vi "Get Array Element Offsets.vi"(8 "error in (no error)":errorcluster, 9 "Max Index":i32=2147483647, 10 "Offset":i32, 11 "JSON":string) -> (0 "error out":errorcluster, 1 "Elements":T2(array[cluster]), 2 "Offset past Array":i32)   [LabVIEW 2017, in "JSONtext.lvlib"]
uses:
  JSONtext.lvlib
  Parsing/Parsing State.ctl
  Parsing/Advance past String.vi
  Parsing/Advance past Number.vi
  Parsing/Advance past Object.vi
  Parsing/Advance past Array.vi
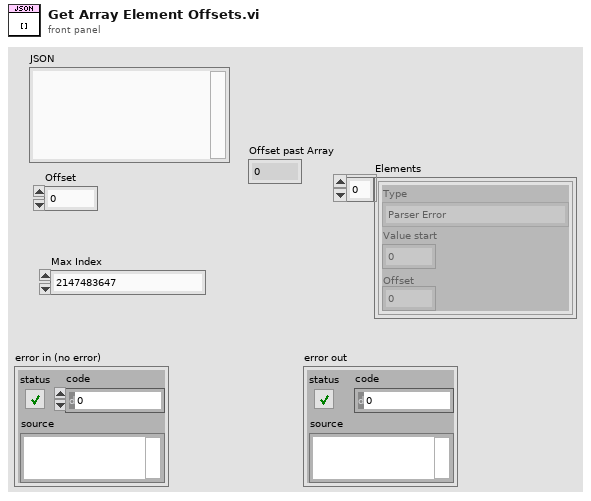
[diagram p1: front panel]
types:
  T1 = typedef "JSONtext.lvlib/Parsing State.ctl" = enum16{"Parser Error", "Object", "Array", "String", "Number/Other", "Leading Whitespace", "Object end", "Array end", "Value end"}
  T2 = cluster{"Type":T1, "Value start":i32, "Offset":i32}[]
  T3 = cluster{"Type":T1, "Value start":i32, "Offset":i32}
  T4 = cluster{"State":T1, "Value start":i32, "index":i32}
  T5 = cluster{"State":T1, "Value start":i32, "index":i32}[]
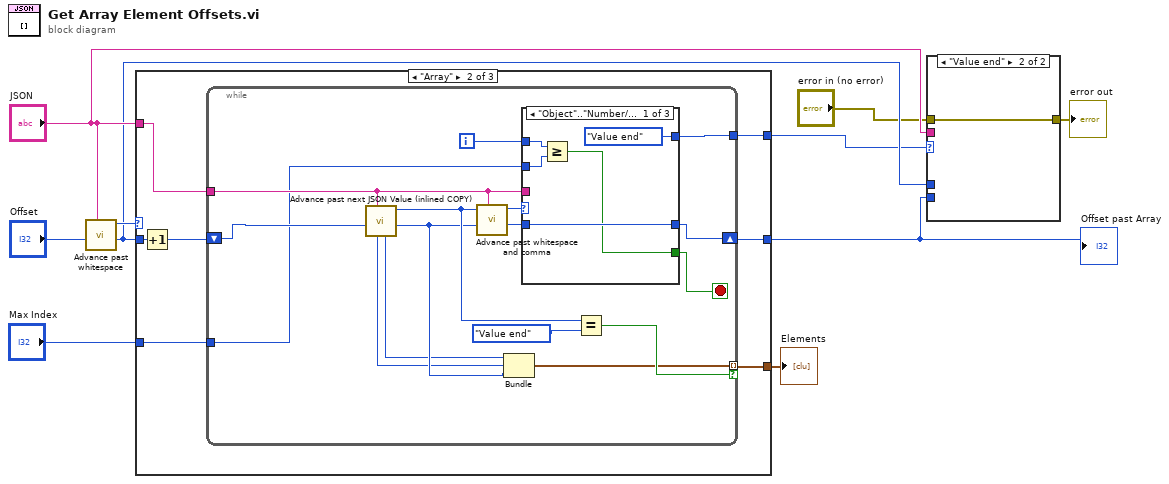
[diagram p0: block diagram]
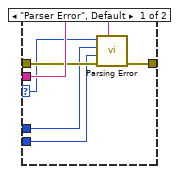
[diagram p2: hidden frame]
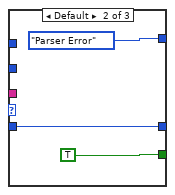
[diagram p4: hidden frame]
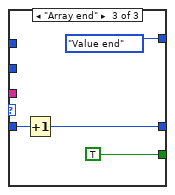
[diagram p5: hidden frame]
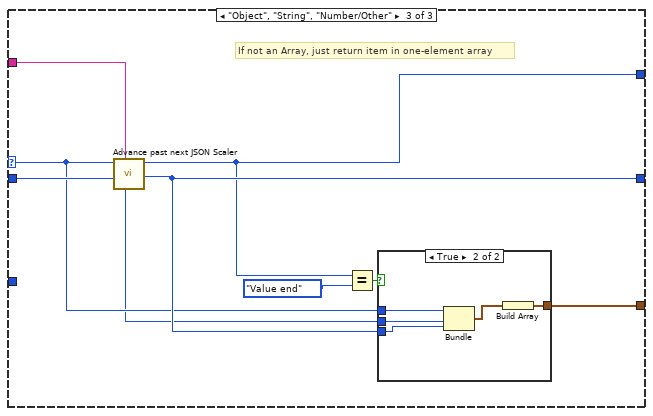
[diagram p6: hidden frame]
diagram:
  n1 = call "Advance past whitespace.vi"("JSON"="JSON", "Offset"="Offset") -> ("Offset of first non-whitespace"=w7:i32, "Parser State"=w9:T1)  [unwired: 8 in]
  n2 = case shown="\"Array\"" w9 {
    selector: w9 -> [w12 _ w50]
    tunnel: [w12 w19 w52] -> w3
    tunnel: [w11 w18 w54] -> w6
    tunnel: [_ w16 w49] -> w2
    tunnel: "JSON" -> [_ w15 w53]
    tunnel: w7 -> [w11 w14 w56]
    tunnel: "Max Index" -> [_ w13 _]
    frame "Parser Error", Default {
    }
    frame "Array" {
      n3 = Increment(x=w14) -> (x+1=w17:i32)
      n4 = while {
        tunnel: w15 -> [w29]
        shift-right: [w32] -> w18
        shift-left: w17 -> [w33]
        tunnel: [w30] -> w19
        tunnel: [w23] -> w16 mode=indexing if=w26
        tunnel: w13 -> [w20]
        i -> [w21]
        stop <- w31 stop-if-true
        n5 = call "Advance past next JSON Value (inlined COPY).vi"("JSON"=w29, "Offset"=w33) -> ("Offset"=w25:i32, "State"=w27:T1, "Type"=w24:T1, "Value start"=w22:i32)  [unwired: 5 in, 1 out]
        n6 = call "Advance past whitespace and comma.vi"("JSON"=w29, "Offset"=w25, "State in"=w27) -> ("Offset past match"=w35:i32, "State"=w34:T1)  [unwired: 7 in]
        n7 = Bundle("Type"=w24, "Value start"=w22, "Offset"=w25) -> (w23:T3)  [unwired: 1 in]
        n8 = case shown="\"Object\"..\"Number/Other\"" w34 {
          tunnel: [w37 TRUE TRUE] -> w31
          tunnel: [Parsing_State."Value end" Parsing_State."Parser Error" Parsing_State."Value end"] -> w30
          tunnel: w35 -> [w40 w41 w45]
          tunnel: [w40 w41 w44] -> w32
          tunnel: w29 -> [_ _ _]
          tunnel: w21 -> [w38 _ _]
          tunnel: w20 -> [w39 _ _]
          frame "Object".."Number/Other" {
            n9 = Greater Or Equal?(x=w38, y=w39) -> (x >= y?=w37:bool)
          }
          frame Default {
          }
          frame "Array end" {
            n10 = Increment(x=w45) -> (x+1=w44:i32)
          }
        }
        n11 = Equal?(x=w27, y=Parsing_State."Value end") -> (x = y?=w26:bool)
      }
    }
    frame "Object", "String", "Number/Other" {
      # "If not an Array, just return item in one-element array"
      n12 = call "Advance past next JSON Scaler.vi"("JSON"=w53, "Offset"=w56, "Parser State in"=w50) -> ("index"=w54:i32, "Parser State"=w52:T1, "Value start"=w48:i32)  [unwired: 6 in]
      n13 = Equal?(x=w52, y=Parsing_State."Value end") -> (x = y?=w51:bool)
      n14 = case shown="True" w51 {
        tunnel: w48 -> [_ w59]
        tunnel: w54 -> [_ w60]
        tunnel: [_ w61] -> w49
        tunnel: w50 -> [_ w58]
        frame False {
        }
        frame True {
          n15 = Bundle("State"=w58, "Value start"=w59, "index"=w60) -> (w57:T4)  [unwired: 1 in]
          n16 = Build Array(w57) -> (w61:T5)
        }
      }
    }
  }
  "Offset past Array" <- w6
  "Elements" <- w2
  n17 = case shown="\"Value end\"" w3 {
    selector: w3 -> [w62 _]
    tunnel: "JSON" -> [w67 _]
    tunnel: "error in (no error)" -> [w66 w68]
    tunnel: [w65 w68] -> w5
    tunnel: w7 -> [w64 _]
    tunnel: w6 -> [w63 _]
    frame "Parser Error", Default {
      n18 = call "Parsing Error.vi"("JSON"=w67, "error in (no error)"=w66, "Offset past match"=w63, "Value start"=w64, "State"=w62) -> ("error out"=w65:errorcluster)  [unwired: 6 in]
    }
    frame "Value end" {
    }
  }
  "error out" <- w5
